vi "Design Challenge Wen.vi"() -> ()   [LabVIEW 2025]
panel:
  in  "stop":bool
  in  "Clear":bool
  in  "Run":bool
  out "XY Graph":cluster{"X":dbl, "Y":dbl}[](graph)
  out "Initial Speed (m/s)":dbl(knob) scale=0.0..25.0
  in  "Angle (theta)":dbl(knob) scale=0.0..89.0
  in  "Mass of my chudd life (kg)":dbl
  in  "Initial Height (m)":dbl
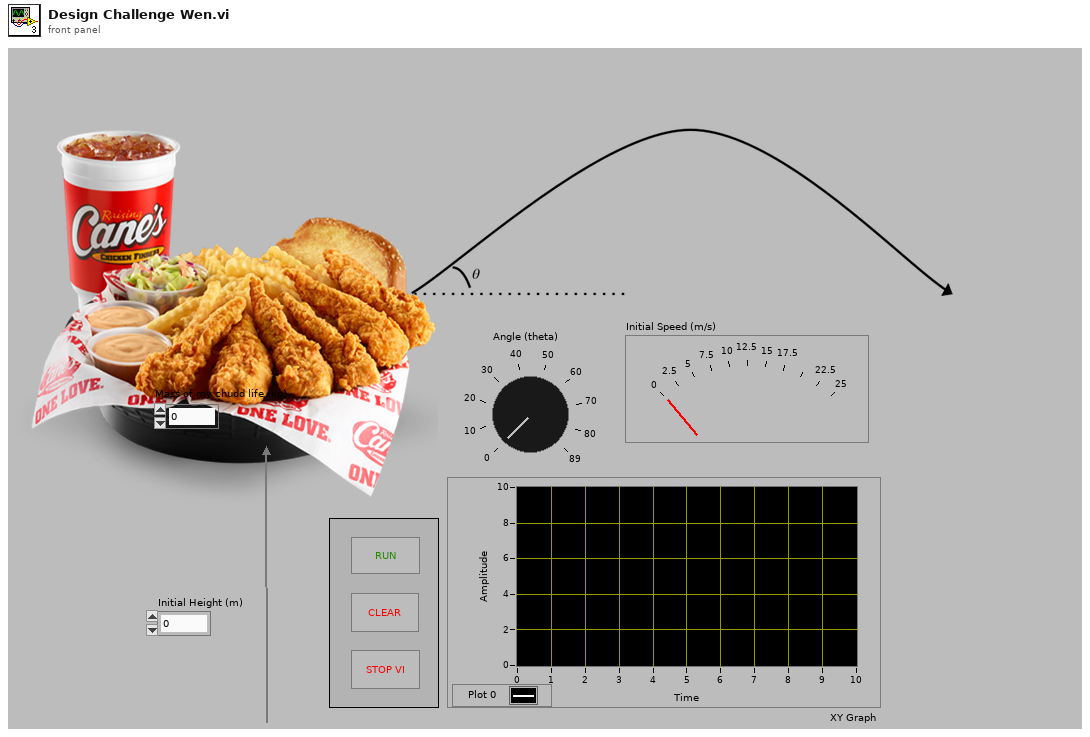
[diagram p1: front panel]
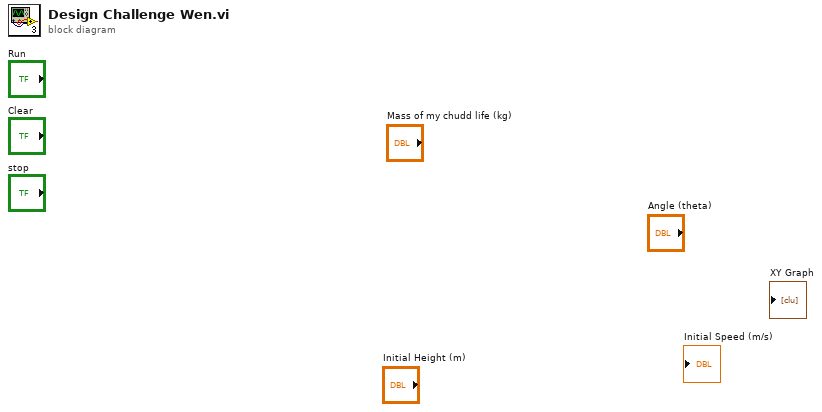
[diagram p0: block diagram]
diagram:
